vi "PyrometrysubVI_irradiance - Copy.vi"(2 "Wavelength Difference (nm)":dbl, 3 "Wavelength in":dbl[](array[numeric]), 4 "Data In":dbl[](array[numeric])) -> (0 "wl out":dbl[](array[numeric]), 1 "FT":dbl[](array[numeric]))   [LabVIEW 2017]
uses:
  <vilib>/Analysis/baseanly.llb/Mean (DBL).vi
  <vilib>/Analysis/NI_AALBase.lvlib
panel:
  in  "Integration time\n(us)":i32=10000
  in  "Pixel Index (Max)":i32=10000
  in  "Pixel Index (Min)":i32=10000
  in  "Pixel Length":i32=10000
  in  "Pixel Index":i32=10000
  in  "Every N pixel":i32=10000
  out "min value 2":dbl
  out "max value 2":dbl
  in  "Fit irradiance":bool
  out "variance":dbl format="%0.2f"
  out "standard deviation":dbl format="%0.2f"
  out "Thermometer":dbl(slide) scale=1000.0..5000.0
  out "Mean background":dbl format="%0.2f"
  out "Average Color temperature \n(Kelvin)":dbl format="%0.2f"
  out "2 color temperature":cluster{"Y":dbl[], "Y":dbl[]}[](graph)
  out "Absolute Irradiance":cluster{"Y":dbl[], "Y":dbl[]}[](graph)
  # "1. Type in file name and file location for raw data saving.\n2. Setup Spectrometer index  (use GetSerialNumber.vi to identify spectrometer index)\n(you only want to connect the Flame-S spectrometer, otherwise, you need to rewrite the calibration subVI.)\n3. Setup integration time and Number of Scan Average.\n(you only can choose integration from 10ms, 20 ms, 100 ms, 200 ms - 1000 ms)\n4. Make sure spectrometerIndex \n5. optionally, adjust wavelengthdifference (# of pixel difference)"
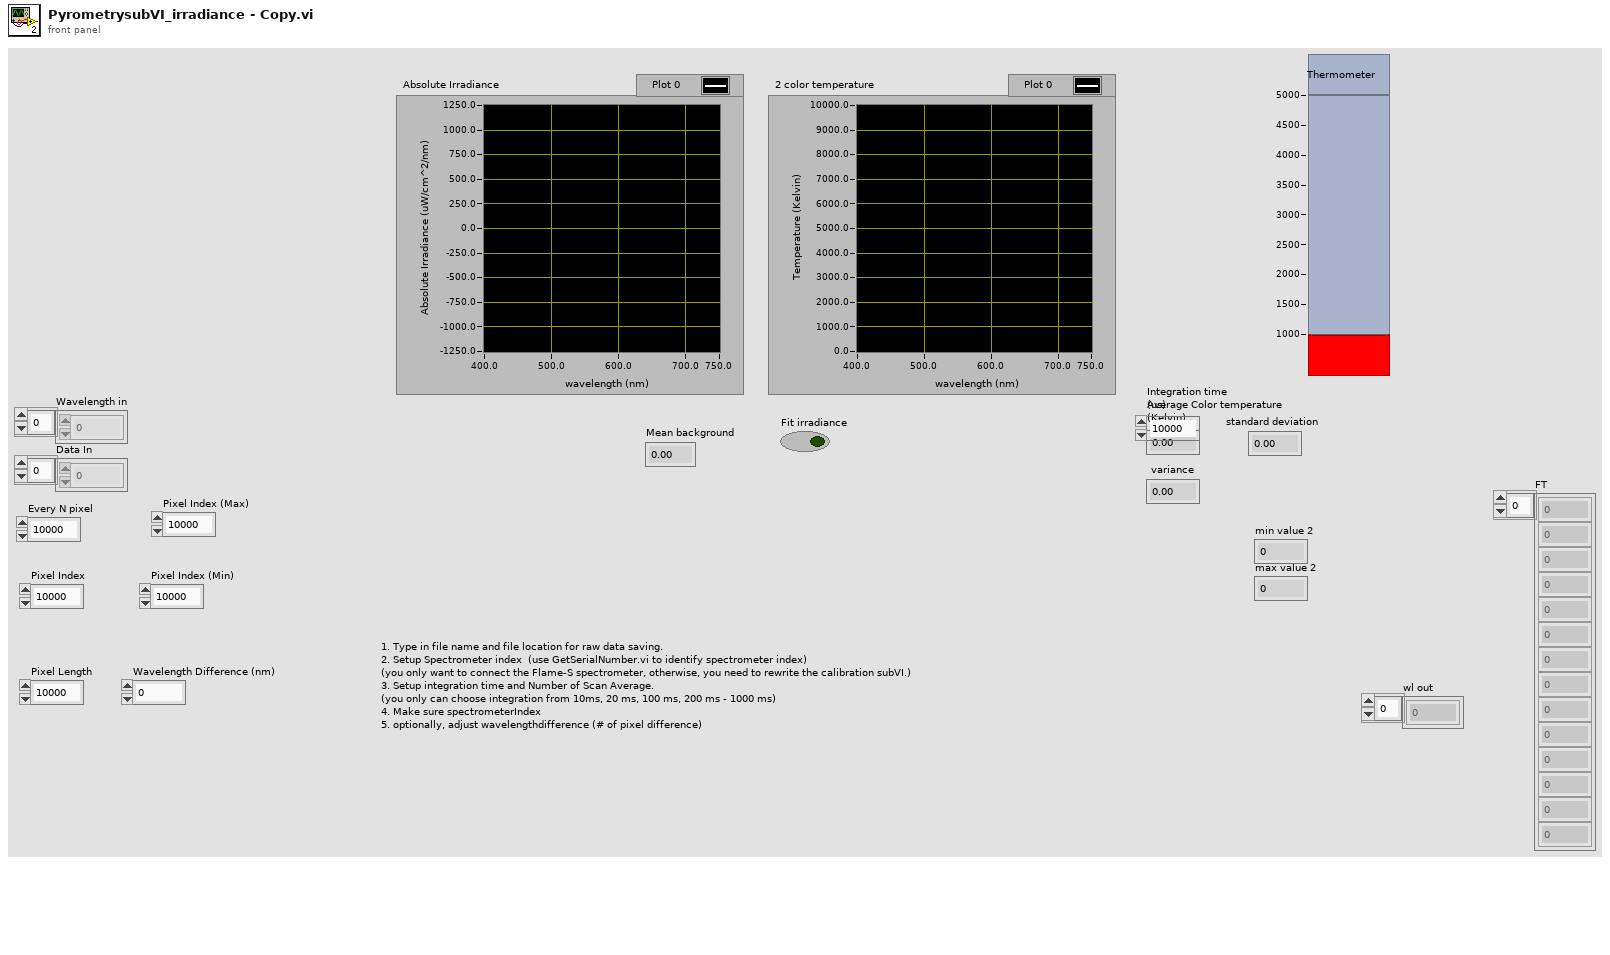
[diagram p1: front panel]
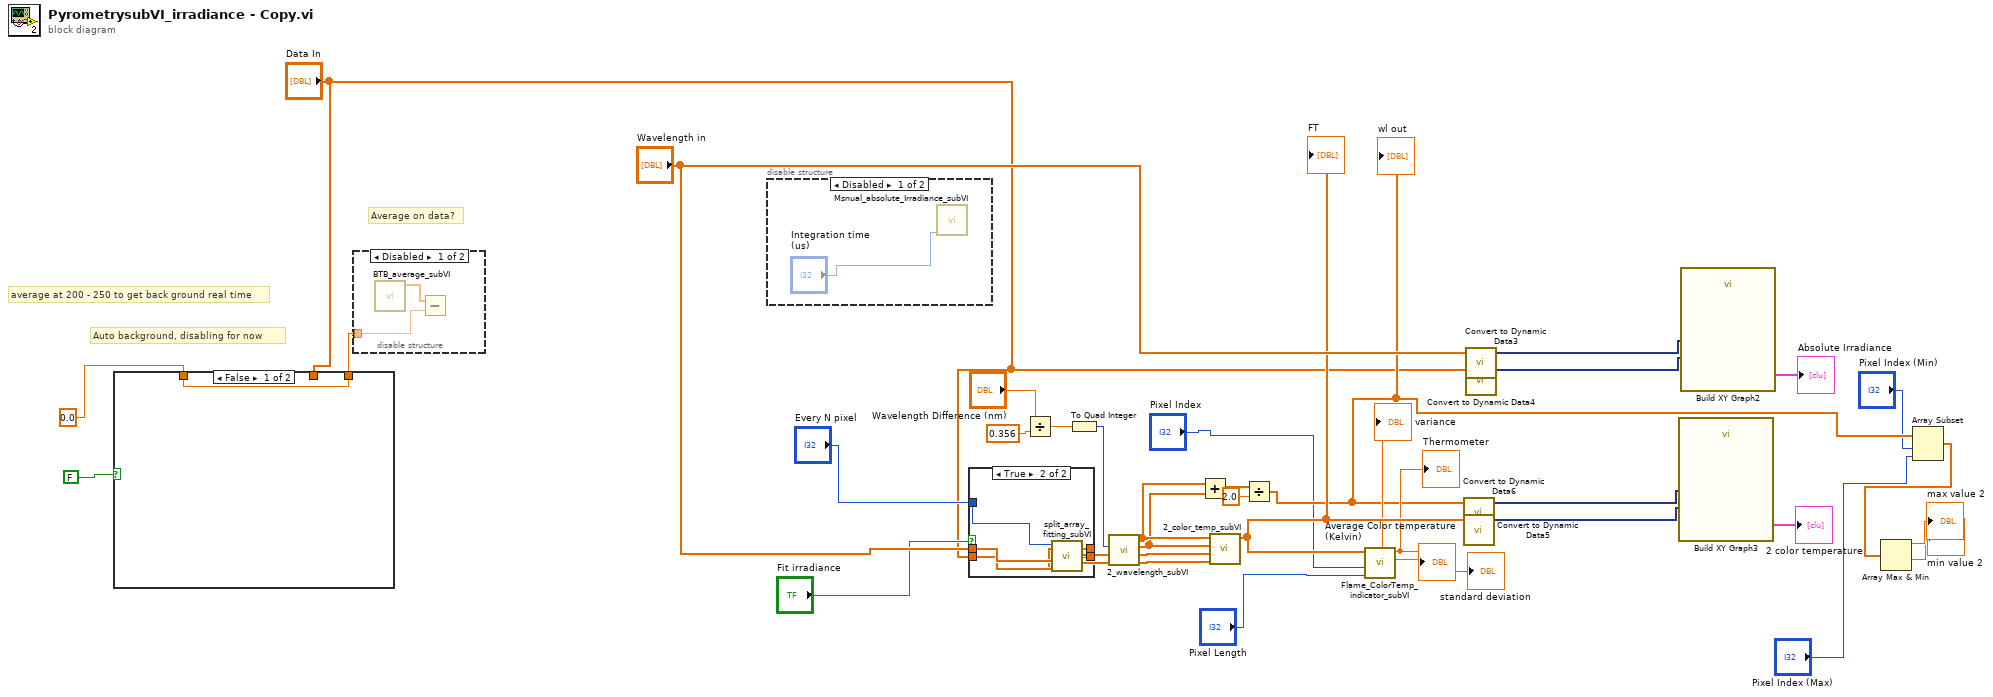
[diagram p0: block diagram]
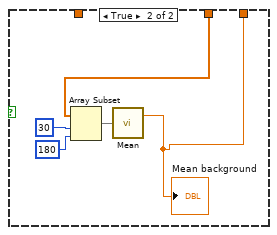
[diagram p5: hidden frame]
diagram:
  # "Average on data?"
  # "Auto background, disabling for now"
  # "average at 200 - 250 to get back ground real time"
  n1 = case shown="False" FALSE ("auto \nback ground") {
    tunnel: "Data In" -> [_ w40]
    tunnel: 0.0 ("manual noise level") -> [w38 _]
    tunnel: [w38 w39] -> w2
    frame False {
    }
    frame True {
      n2 = Array Subset(array=w40, index=30, length=180) -> (w43:dbl[])
      n3 = call-poly <vilib>:"Mean.vi"("X"=w43) -> ("mean"=w39:dbl)  [unwired: 1 out]
      "Mean background" <- w39
    }
  }
  n4 = disable-structure shown="Disabled" {
    disable-tunnel: w2 -> [w44 _]
    frame Disabled {
      n5 = call "BTB_average_subVI.vi"() -> ("Array"=w45:dbl[])  [unwired: 11 in]
      n6 = Subtract(x=w45, y=w44) -> ()  [unwired: 1 out]
    }
    frame Enabled {
    }
  }
  n7 = disable-structure shown="Disabled" {
    frame Disabled {
      n8 = call "Msnual_absolute_Irradiance_subVI.vi"("Integration time\n(us)"="Integration time\n(us)") -> ("Manual_absolute_Irradiance"=w47:dbl[])  [unwired: 9 in, 1 out]
    }
    frame Enabled {
    }
  }
  n9 = case shown="True" "Fit irradiance" {
    tunnel: "Wavelength in" -> [w49 w54]
    tunnel: "Data In" -> [w48 w53]
    tunnel: [w49 w52] -> w21
    tunnel: [w48 w51] -> w20
    tunnel: "Every N pixel" -> [_ w50]
    frame False {
    }
    frame True {
      n10 = call "split_array_fitting_subVI.vi"("irr-irradiance input"=w53, "wl-irradiance input"=w54, "Every N pixel"=w50) -> ("irr-irradiance output"=w51:dbl[], "wl-irradiance output"=w52:dbl[])  [unwired: 5 in]
    }
  }
  n11 = Divide(x="Wavelength Difference (nm)", y=0.356) -> (x/y=w25:dbl)
  n12 = To Quad Integer(1:w25) -> (0:w24:i64)
  n13 = call "2_wavelength_subVI.vi"("Input_Intensity"=w20, "Input_wavelength"=w21, "pixel difference"=w24) -> ("Intensity_2"=w31:dbl[], "Intensity_1"=w32:dbl[], "Wavelength_2"=w16:dbl[], "Wavelength_1"=w17:dbl[])  [unwired: 5 in]
  n14 = Add(x=w17, y=w16) -> (x+y=w19:dbl[])
  n15 = call "2_color_temp_subVI.vi"("E1 2"=w31, "E1"=w32, "In_WL1 2"=w16, "In_WL1"=w17) -> ("FT"=w28:dbl[])  [unwired: 7 in]
  "FT" <- w28
  n16 = Divide(x=w19, y=2.0) -> (x/y=w13:dbl[])
  "wl out" <- w13
  n17 = call "Flame_ColorTemp_indicator_subVI.vi"("pixel length"="Pixel Length", "pixel index"="Pixel Index", "Color Temp"=w28) -> ("variance"=→"variance":dbl, "standard deviation"=→"standard deviation":dbl, "Average Color temperature"=→"Average Color temperature \n(Kelvin)" →"Thermometer":dbl)  [unwired: 6 in]
  n18 = call "Convert to Dynamic Data6"("Array"=w13) -> ("Dynamic Data Type"=w29:dynamicdata)  [unwired: 3 in]
  n19 = call "Convert to Dynamic Data5"("Array"=w28) -> ("Dynamic Data Type"=w30:dynamicdata)  [unwired: 3 in]
  n20 = call "Convert to Dynamic Data3"("Array"="Wavelength in") -> ("Dynamic Data Type"=w35:dynamicdata)  [unwired: 3 in]
  n21 = call "Convert to Dynamic Data4"("Array"="Data In") -> ("Dynamic Data Type"=w34:dynamicdata)  [unwired: 3 in]
  n22 = call "Build XY Graph3"("Y Input"=w30, "X Input"=w29) -> ("XY Graph"=→"2 color temperature":cluster{"X":dbl[], "Y":dbl[]}[])  [unwired: 8 in, 1 out]
  n23 = call "Build XY Graph2"("Y Input"=w34, "X Input"=w35) -> ("XY Graph"=→"Absolute Irradiance":cluster{"X":dbl[], "Y":dbl[]}[])  [unwired: 8 in, 1 out]
  n24 = Array Subset(array=w13, index="Pixel Index (Min)", length="Pixel Index (Max)") -> (w12:dbl[])
  n25 = Array Max & Min(array=w12) -> (max value=→"max value 2":dbl, min value=→"min value 2":dbl)  [unwired: 2 out]
